vi "TDMS_数据读取.vi"(5 "总数（-1:全部）":i64=600, 7 "偏移量(0)":i64, 8 "error in (no error)":errorcluster caption="错误输入（无错误）", 9 "CH Name[]":string, 10 "组名称":string, 11 "tdms文件":refnum<k34>) -> (0 "error out":errorcluster caption="错误输出", 1 "X标尺":cluster{"Max":dbl, "Min":dbl} {"Min" format="%#_6f"; "Max" format="%#.10f"}, 2 "曲线":cluster{"时间":dbl[], "曲线":dbl[]}, 3 "tdms文件 2":refnum<k34>, 4 "Y标尺":cluster{"Max":dbl, "Min":dbl})   [LabVIEW 2018]
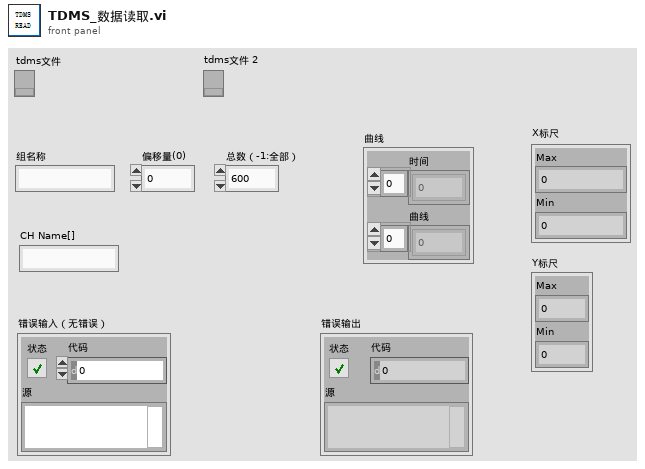
[diagram p1: front panel]
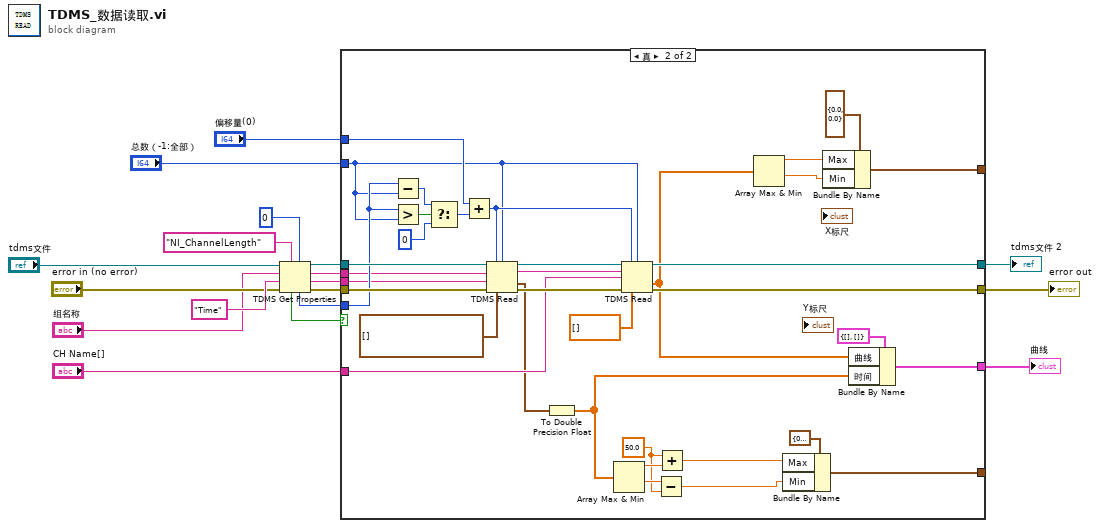
[diagram p0: block diagram]
diagram:
  n1 = TDMS Get Properties(5:i64 0, 7:"NI_ChannelLength" ("channel name(s) in"), 8:"error in (no error)", 9:"Time" ("通道名称"), 10:"组名称", 11:"tdms文件") -> (0:w14:errorcluster, 1:w11:string, 2:w12:string, 3:w13:refnum<k34>, 4:w15:i64, 6:w16:bool)
  n2 = case shown="真" w16 {
    tunnel: w15 -> [_ w51]
    tunnel: w14 -> [w20 w53]
    tunnel: w13 -> [w19 w54]
    tunnel: w12 -> [_ w50]
    tunnel: w11 -> [_ w49]
    tunnel: "CH Name[]" -> [_ w27]
    tunnel: [_ w44] -> w1
    tunnel: [w20 w43] -> w5
    tunnel: [w19 w42] -> w3
    tunnel: "总数（-1:全部）" -> [_ w21]
    tunnel: "偏移量(0)" -> [_ w39]
    tunnel: [_ w33] -> _
    tunnel: [_ w23] -> _
    frame False {
    }
    frame True {
      w30 = 50.0 ("x")
      n3 = Subtract(x=w51, y=w21) -> (x-y=w52:i64)
      n4 = Greater?(x=w51, y=w21) -> (0:w55:bool)
      n5 = Select(t=w52, s=w55, f=i64 0 ("偏移量(0)")) -> (s? t:f=w40:i64)
      n6 = Add(x=w39, y=w40) -> (x+y=w41:i64)
      n7 = TDMS Read(0:w54, 1:w41, 2:w21, 5:w50, 7:w49, 11:w53, 12:timestamp[] [] ("当前时间")) -> (4:w48:refnum<k34>, 6:w47:string, 10:w25:timestamp[], 15:w46:errorcluster)  [unwired: 1 in, 2 out]
      n8 = To Double Precision Float(number=w25) -> (double precision float=w24:dbl[])
      n9 = Array Max & Min(array=w24) -> (max value=w32:dbl, min value=w31:dbl)  [unwired: 2 out]
      n10 = TDMS Read(0:w48, 1:w41, 2:w21, 5:w47, 7:w27, 11:w46, 12:dbl[] []) -> (4:w42:refnum<k34>, 10:w34:dbl[], 15:w43:errorcluster)  [unwired: 1 in, 3 out]
      n11 = Subtract(x=w31, y=w30) -> (x-y=w28:dbl)
      n12 = Add(x=w30, y=w32) -> (x+y=w29:dbl)
      n13 = Array Max & Min(array=w34) -> (max value=w36:dbl, min value=w37:dbl)  [unwired: 2 out]
      n14 = Bundle By Name(cluster=cluster{"Max":dbl, "Min":dbl} {"Max"=0.0, "Min"=0.0} ("X标尺"), "Max"=w29, "Min"=w28) -> (w23:cluster{"Max":dbl, "Min":dbl})
      n15 = Bundle By Name(cluster=cluster{"Max":dbl, "Min":dbl} {"Max"=0.0, "Min"=0.0} ("Y标尺"), "Max"=w36, "Min"=w37) -> (w33:cluster{"Max":dbl, "Min":dbl})
      n16 = Bundle By Name(cluster=cluster{"时间":dbl[], "曲线":dbl[]} {"时间"=[], "曲线"=[]}, "曲线"=w34, "时间"=w24) -> (w44:cluster{"时间":dbl[], "曲线":dbl[]})
    }
  }
  "tdms文件 2" <- w3
  "error out" <- w5
  "曲线" <- w1
